vi "Timer_GetAttributes.vi"(8 "error in (no error)":errorcluster caption="错误输入（无错误）", 11 "Timer 输入":refnum<class "Timer.lvclass">) -> (0 "error out":errorcluster caption="错误输出", 1 "数据值引用":refnum<data-value>, 2 "attribute":T1, 3 "Timer 输出":refnum<class "Timer.lvclass">)   [LabVIEW 2019, in "Timer.lvclass"]
uses:
  Timer.lvclass
  attribute/Attribute.ctl
  Timer.lvclass/Timer.ctl
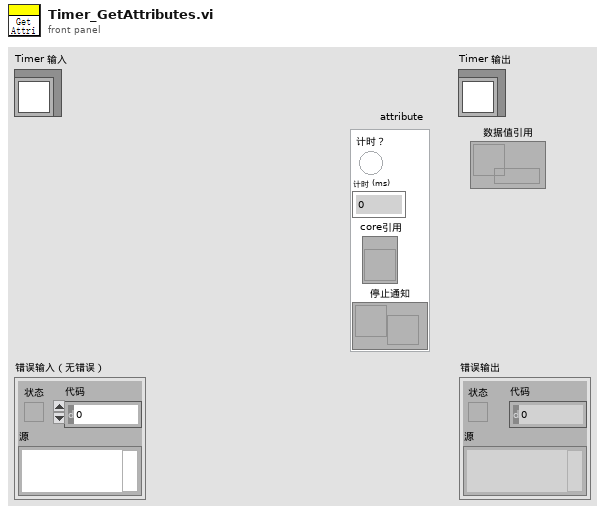
[diagram p1: front panel]
types:
  T1 = typedef "Timer.lvclass/Attribute.ctl" = cluster{"计时？":bool, "计时 (ms)":u32, "core引用":refnum<vi>, "停止通知":refnum<notifier>}
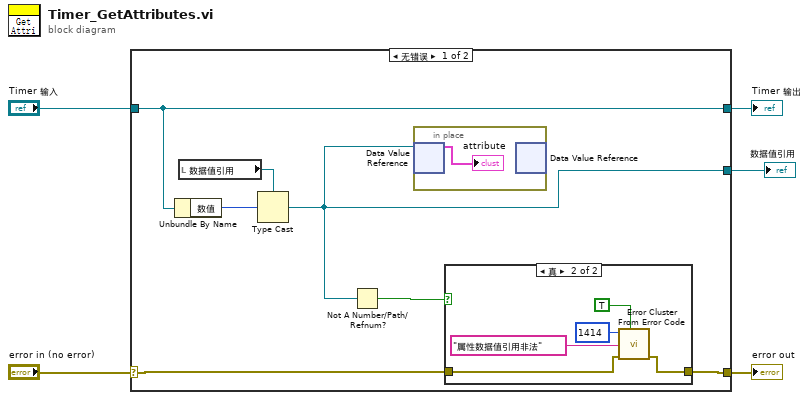
[diagram p0: block diagram]
diagram:
  n1 = case shown="无错误" "error in (no error)" {
    selector: "error in (no error)" -> [w7 w21]
    tunnel: [w8 w21] -> w4
    tunnel: [w12 w20] -> w2
    tunnel: "Timer 输入" -> [w12 w20]
    tunnel: [w6 _] -> w1
    frame No Error {
      n2 = Unbundle By Name(w12) -> ("数值"=w11:u32)
      n3 = local read "数据值引用"() -> (w10:refnum<data-value>)
      n4 = Type Cast(type=w10, x=w11) -> (*(type *) &x=w6:refnum<data-value>)
      n5 = Not A Number/Path/Refnum?(number/path/refnum=w6) -> (NaN/Path/Refnum?=w9:bool)
      n6 = in-place {
        n7 = in-place-dvr #1(w6) -> (→"attribute":T1)  [unwired: 1 out]
        n8 = in-place-dvr #1() -> ()  [unwired: 1 in, 2 out]
      }
      n9 = case shown="真" w9 {
        tunnel: [w14 w18] -> w8
        tunnel: w7 -> [w14 w19]
        frame False {
        }
        frame True {
          n10 = call <vilib>:"Error Cluster From Error Code.vi"("show call chain? (False)"=TRUE, "error in (no error)"=w19, "error message (\"\")"="属性数据值引用非法" ("error message (\"\")"), "error code (0)"=1414) -> ("error out"=w18:errorcluster)  [unwired: 5 in]
        }
      }
    }
    frame Error {
    }
  }
  "error out" <- w4
  "Timer 输出" <- w2
  "数据值引用" <- w1
